vi "Cleanup.vi"(8 "error in (no error)":errorcluster, 11 "ArrayBlank in":refnum<class "ArrayBlank.lvclass">) -> (0 "error out":errorcluster, 3 "ArrayBlank out":refnum<class "ArrayBlank.lvclass">)   [LabVIEW 2018, in "OOPanel.lvlib" / "ArrayBlank.lvclass"]
uses:
  ArrayBlank.lvclass
  Panel/Panel.lvclass
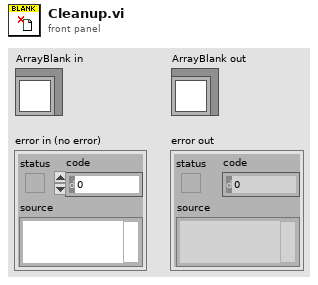
[diagram p1: front panel]
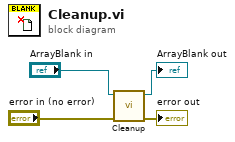
[diagram p0: block diagram]
diagram:
  n1 = call-parent "Cleanup.vi"("error in (no error)"="error in (no error)", "Panel in"="ArrayBlank in") -> ("error out"=→"error out":errorcluster, "Panel out"=→"ArrayBlank out":refnum<class "ArrayBlank.lvclass">)  [unwired: 8 in]
